vi "example_01_load_api.vi"() -> ()   [LabVIEW 2015, in "lv-dialog-interfaces.lvlib" / "v1.lvlib"]
doc: "Use this to load the lv-dialog-interfaces v1 class into memory, keep the VI open to ensure it doesn't get garbage collected."
uses:
  v1.lvlib
  v1.lvclass
  <userlib>/antonio-alexander/lv-dialog/api/v1/public/class/v1.lvclass
  <userlib>/antonio-alexander/lv-dialog/api/v1/public/_subvis/advanced/load_class-class.vi
  <userlib>/antonio-alexander/lv-dialog/api/v1/v1.lvlib
panel:
  out "error out":errorcluster
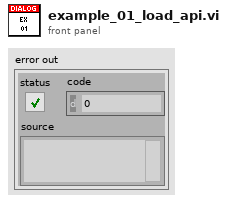
[diagram p1: front panel]
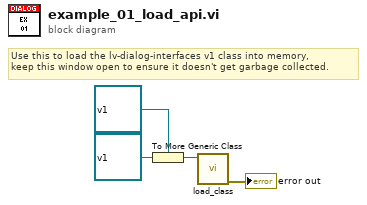
[diagram p0: block diagram]
diagram:
  # "Use this to load the lv-dialog-interfaces v1 class into memory,\nkeep this window open to ensure it doesn't get garbage collected."
  n1 = To More Generic Class(target class=refnum<class "v1.lvclass"> refnum ("class"), reference=refnum<class "v1.lvclass"> refnum ("lv-dialog-interfaces.lvlib:v1.lvclass")) -> (generic class reference=w2:refnum<class "v1.lvclass">)
  n2 = call-poly <userlib>:"load_class.vi"("class"=w2) -> ("error out"=→"error out":errorcluster)  [unwired: 10 in]
